vi "Get Port Incoming and Outgoing Sections.vi"(8 "error in":errorcluster, 11 "Port Ref":T1 format="%.0x") -> (0 "error out":errorcluster, 1 "Outgoing":T1 format="%.0x", 2 "Incoming":T1 format="%.0x", 3 "Port Ref out":T1 format="%.0x")   [LabVIEW 2020, in "Communication Bus Template Scripting.lvlib"]
uses:
  <vilib>/NI VeriStand/Custom Device API/Custom Device Item Ref.ctl
  Constants.vi
  Communication Bus Template Scripting.lvlib
  <vilib>/NI VeriStand/Custom Device Tools/Custom Device Utility Library/Custom Device Utility Library.lvlib
  <vilib>/NI VeriStand/Custom Device Tools/Custom Device Utility Library/NI VeriStand - Search for Item by GUID.vi
  <vilib>/NI VeriStand/Custom Device API/Custom Device API.lvlib
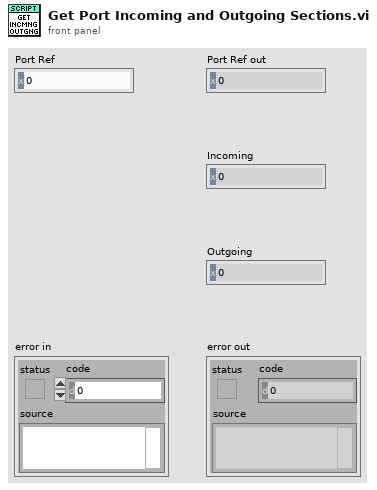
[diagram p1: front panel]
types:
  T1 = typedef "Custom Device API.lvlib/Custom Device Item Ref.ctl" = u64
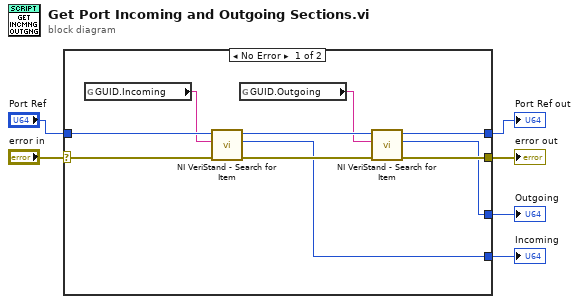
[diagram p0: block diagram]
diagram:
  n1 = case shown="No Error" "error in" {
    selector: "error in" -> [w13 w18]
    tunnel: "Port Ref" -> [w16 w17]
    tunnel: [w11 w18] -> w5
    tunnel: [w14 w17] -> w4
    tunnel: [w8 _] -> w2
    tunnel: [w7 _] -> w1
    frame No Error {
      n2 = global read "Constants.vi" "GUID.Incoming"() -> (w9:string)
      n3 = call-poly <vilib>:"NI VeriStand - Search for Item.vi"("error in"=w13, "Item GUID"=w9, "Section Ref in"=w16) -> ("error out"=w12:errorcluster, "Item Ref"=w7:T1, "Section Ref out"=w15:T1)  [unwired: 5 in, 1 out]
      n4 = global read "Constants.vi" "GUID.Outgoing"() -> (w10:string)
      n5 = call-poly <vilib>:"NI VeriStand - Search for Item.vi"("error in"=w12, "Item GUID"=w10, "Section Ref in"=w15) -> ("error out"=w11:errorcluster, "Item Ref"=w8:T1, "Section Ref out"=w14:T1)  [unwired: 5 in, 1 out]
    }
    frame Error {
    }
  }
  "error out" <- w5
  "Port Ref out" <- w4
  "Outgoing" <- w2
  "Incoming" <- w1
